vi "destroyModuleManager.vi"(7 "path in":path=path "C:/dev/Hexagon-VTD-Custom-Device/Libraries/VC.dll", 8 "error in (no error)":errorcluster, 11 "mmHandle":u64) -> (0 "error out":errorcluster)   [LabVIEW 2023, in "MM.lvlib"]
uses:
  MM.lvlib
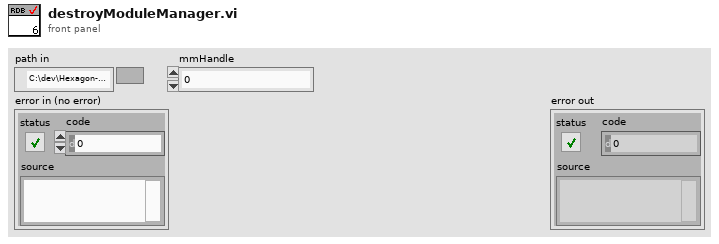
[diagram p1: front panel]
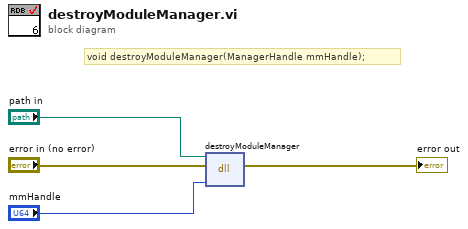
[diagram p0: block diagram]
diagram:
  # "void destroyModuleManager(ManagerHandle mmHandle);"
  n1 = dll-call lib="C:/dev/Hexagon-VTD-Custom-Device/Libraries/libMM.dll" fn="destroyModuleManager"(path in="path in", error in="error in (no error)", "mmHandle"="mmHandle") -> (error out=→"error out":errorcluster)  [unwired: 3 in, 1 out]
